vi "SV TDMS Write XY (N Ch).vi"(0 "tdms file":refnum<k34>, 2 "write mode":u16(ring) items=["Append", "New group", "Overwrite"], 5 "group name in":string="XY", 7 "channel names in":string[](array[string]), 9 "XY":cluster{"X":dbl[], "Y":dbl[]}[](array[cluster]), 11 "error in":errorcluster, 12 "unit info":T5, 13 "function info":T4={"function type"=0, "function subtype"=2, "X-domain"=0} {"X-domain" items=["Time (s)"=0, "Frequency-CB (Hz)"=1, "Frequency-CPB (Hz)"=1248, "Frequency-Arbitrary (Hz)"=2357, "Quefrency (s)"=2, "Revolutions (rev)"=3, "Order"=4, "Speed (RPM)"=11, "Speed (rad/s)"=21, "Index"=65535]; "function subtype" items=["Unscaled binary"=0, "Scaled voltage"=1, "Scaled engineering units"=2, "-"=10, "Value"=19, "DC"=11, "AC"=12, "RMS^2"=13, "RMS"=14, "Peak"=15, "Peak to peak"=16, "-"=20, "1/1 octave"=21, "1/3 octave"=22, "1/6 octave"=23, "1/12 octave"=24, "1/24 octave"=25, "-"=30, "Density"=31, "Magnitude"=32, "Phase"=33, "Real"=34, "Imaginary"=35, "Complex"=345, "Coherence"=36, "-"=90, "Unknown"=99]; "function type" items=["Signal"=0, "Speed"=3, "Ratio"=6, "Count"=7, "-"=9, "Level"=10, "-"=19, "Octave Spectrum"=20, "-"=29, "FFT Auto Spectrum"=30, "FFT Cross Spectrum"=40, "Frequency Response"=50, "-"=59, "Event"=90]}) -> (4 "tdms file out":refnum<k34>, 6 "group name out":string, 8 "channel names out":string[](array[string]), 15 "error out":errorcluster)   [LabVIEW 2017]
uses:
  <vilib>/addons/_NISVFA/_Shared subVIs/Controls/NI Function Type.ctl
  <vilib>/addons/_NISVFA/_Shared subVIs/Controls/NI Function SubType.ctl
  <vilib>/addons/_NISVFA/_Shared subVIs/Controls/svc_X-Axis Units.ctl
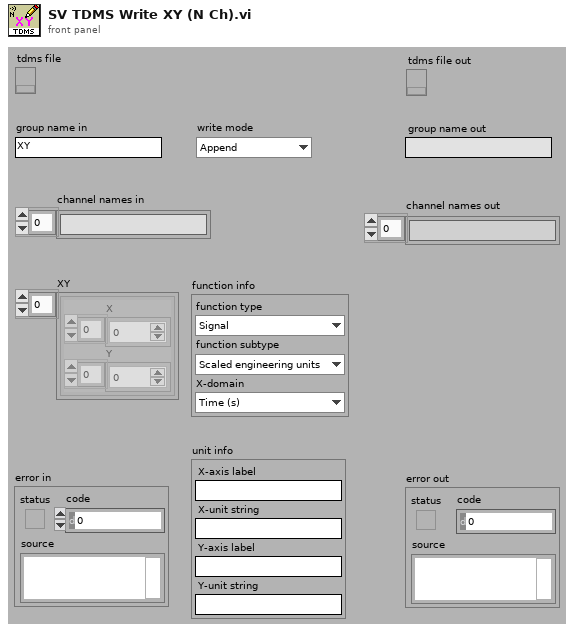
[diagram p1: front panel]
types:
  T1 = typedef "NI Function Type.ctl" = u16
  T2 = typedef "NI Function SubType.ctl" = u16
  T3 = typedef "svc_X-Axis Units.ctl" = u16
  T4 = cluster{"function type":T1, "function subtype":T2, "X-domain":T3}
  T5 = cluster{"X-axis label":string, "X-unit string":string, "Y-axis label":string, "Y-unit string":string}
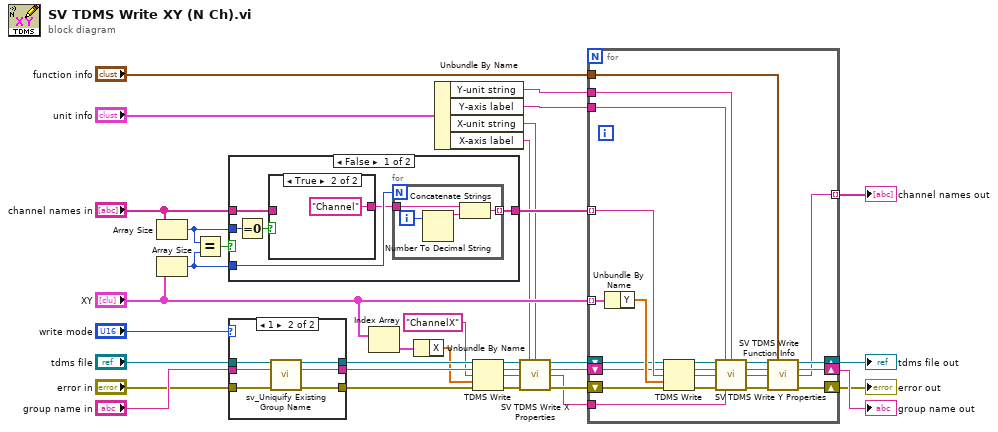
[diagram p0: block diagram]
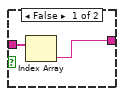
[diagram p2: hidden frame]
diagram:
  n1 = Array Size(array="channel names in") -> (size(s)=w17:i32)
  n2 = Array Size(array="XY") -> (size(s)=w16:i32)
  n3 = Equal?(x=w17, y=w16) -> (x = y?=w20:bool)
  n4 = case shown="False" w20 {
    tunnel: "channel names in" -> [w38 w48]
    tunnel: [w35 w48] -> w18
    tunnel: w17 -> [w40 _]
    tunnel: w16 -> [w37 _]
    frame False {
      n5 = Equal To 0?(x=w40) -> (x = 0?=w39:bool)
      n6 = case shown="True" w39 {
        tunnel: w38 -> [w46 _]
        tunnel: [w45 "Channel" ("channel name")] -> w36
        frame False {
          n7 = Index Array(array=w46) -> (element=w45:string)  [unwired: 1 in]
        }
        frame True {
        }
      }
      n8 = for {
        N: w37 -> [_]
        tunnel: w36 -> [w42]
        tunnel: [w41] -> w35 mode=indexing
        i -> [w43]
        n9 = Number To Decimal String(number=w43) -> (decimal integer string=w44:string)  [unwired: 1 in]
        n10 = Concatenate Strings(w42, w44) -> (w41:string)
      }
    }
    frame True {
    }
  }
  n11 = case shown="1" "write mode" {
    tunnel: [w51 w52] -> w34
    tunnel: [w49 w54] -> w33
    tunnel: "group name in" -> [w49 w55]
    tunnel: [w50 w53] -> w31
    tunnel: "error in" -> [w50 w56]
    tunnel: "tdms file" -> [w51 w57]
    frame 0, Default {
    }
    frame 1 {
      n12 = call <vilib>:"sv_Uniquify Existing Group Name.vi"("tdms file ref"=w57, "group name"=w55, "error in"=w56) -> ("tdms file out"=w52:refnum<k34>, "unique group"=w54:string, "error out"=w53:errorcluster)  [unwired: 10 in]
    }
  }
  n13 = Index Array(array="XY") -> (element=w22:cluster{"X":dbl[], "Y":dbl[]})  [unwired: 1 in]
  n14 = Unbundle By Name(w22) -> ("X"=w23:dbl[])
  n15 = Unbundle By Name("unit info") -> ("Y-unit string"=w26:string, "Y-axis label"=w25:string, "X-unit string"=w9:string, "X-axis label"=w10:string)
  n16 = TDMS Write(0:w34, 5:w33, 7:"ChannelX" ("channel name(s) in (Untitled)"), 9:w23, 11:w31) -> (4:w14:refnum<k34>, 6:w13:string, 8:w12:string, 15:w11:errorcluster)  [unwired: 1 in]
  n17 = call <vilib>:"SV TDMS Write X Properties.vi"("tdms file in"=w14, "X-axis label"=w10, "X-unit string"=w9, "group name"=w13, "channel name"=w12, "error in"=w11) -> ("tdms file out"=w8:refnum<k34>, "group name"=w7:string, "channel name"=w4:string, "error out"=w6:errorcluster)  [unwired: 6 in]
  n18 = for {
    tunnel: w26 -> [w68]
    tunnel: w25 -> [w69]
    tunnel: w18 -> [w77] mode=indexing
    shift-right: [w60] -> w2
    shift-left: w8 -> [w75]
    shift-right: [w61] -> w28
    shift-left: w7 -> [w76]
    shift-right: [w58] -> w1
    shift-left: w6 -> [w74]
    tunnel: "XY" -> [w79] mode=indexing
    tunnel: "function info" -> [w67]
    tunnel: w4 -> [w62]
    tunnel: [w59] -> w3 mode=indexing
    n19 = Unbundle By Name(w79) -> ("Y"=w78:dbl[])
    n20 = TDMS Write(0:w75, 5:w76, 7:w77, 9:w78, 11:w74) -> (4:w73:refnum<k34>, 6:w72:string, 8:w71:string, 15:w70:errorcluster)  [unwired: 1 in]
    n21 = call <vilib>:"SV TDMS Write Y Properties.vi"("tdms file"=w73, "y-axis label"=w69, "y-unit string"=w68, "group name"=w72, "channel name"=w71, "error in (no error)"=w70, "xchannel name"=w62) -> ("tdms file out"=w66:refnum<k34>, "group name"=w65:string, "channel name"=w64:string, "error out"=w63:errorcluster)  [unwired: 5 in]
    n22 = call <vilib>:"SV TDMS Write Function Info.vi"("tdms file in"=w66, "function info"=w67, "group name"=w65, "channel name"=w64, "error in (no error)"=w63) -> ("tdms file out"=w60:refnum<k34>, "group name out"=w61:string, "channel name out"=w59:string, "error out"=w58:errorcluster)  [unwired: 7 in]
  }
  "error out" <- w1
  "tdms file out" <- w2
  "group name out" <- w28
  "channel names out" <- w3
